vi "SE_E5_Práctica3.vi"() -> ()   [LabVIEW 2015]
uses:
  <vilib>/myRIO/Instrument Drivers/Onboard IO/DIO/typedefs/DIO Reference.ctl
  <vilib>/myRIO/Common/Instrument Driver Framework/Utilities/typedefs/myRIO Generic Hardware Reference.ctl
  <vilib>/myRIO/Common/Instrument Driver Framework/Utilities/typedefs/Hardware Version Enum.ctl
  <vilib>/myRIO/Common/Instrument Driver Framework/Utilities/typedefs/myRIO v1.0 Reference.ctl
  <vilib>/myRIO/Common/Instrument Driver Framework/Utilities/typedefs/Generic FPGA Reference.ctl
  <vilib>/myRIO/Common/Instrument Driver Framework/myRIO v1.0/DIO/typedefs/DIO Channels List.ctl
  <vilib>/myRIO/Common/Instrument Driver Framework/myRIO v1.0/DIO/typedefs/DIO Channels Enum.ctl
  <vilib>/userdefined/High Color/nirio_resource_hc.ctl
  <vilib>/myRIO/Common/Instrument Driver Framework/Utilities/vis/Is FPGA Ref Available.vi
  <vilib>/myRIO/Common/Instrument Driver Framework/myRIO v1.0/DIO/vis/myRIO v1.1 Open DIO.vi
  <vilib>/myRIO/Instrument Drivers/Onboard IO/DIO/vis/Read.vi
  <vilib>/myRIO/Common/Instrument Driver Framework/Utilities/vis/Validate Channels.vi
  <vilib>/myRIO/Common/Instrument Driver Framework/myRIO v1.0/DIO/vis/myRIO v1.0 Reserve DIO.vi
  <vilib>/myRIO/Common/Instrument Driver Framework/myRIO v1.0/Resource Manager/vis/myRIO v1.0 Reserve Channel List.vi
  <vilib>/myRIO/Common/Instrument Driver Framework/myRIO v1.0/DIO/vis/myRIO v1.0 Build MUX Configuration DIO.vi
  <vilib>/myRIO/Common/Instrument Driver Framework/myRIO v1.0/Resource Manager/vis/myRIO v1.0 Reserve Channel.vi
  <vilib>/myRIO/Common/Instrument Driver Framework/myRIO v1.0/Resource Manager/vis/myRIO v1.0 Unreserve Channel.vi
  <vilib>/myRIO/Common/Instrument Driver Framework/myRIO v1.0/Resource Manager/vis/myRIO v1.0 Create Configuration List.vi
  <vilib>/myRIO/Common/Instrument Driver Framework/myRIO v1.0/Resource Manager/vis/myRIO v1.0 Build Mutex Name.vi
  <vilib>/Utility/VariantDataType/GetNumericInfo.vi
  <vilib>/Utility/error.llb/Error Cluster From Error Code.vi
  <vilib>/myRIO/Common/Instrument Driver Framework/myRIO v1.0/myRIO v1.1 Open.vi
  <vilib>/myRIO/Common/Instrument Driver Framework/Utilities/vis/IO Manager.vi
  <vilib>/myRIO/Common/Instrument Driver Framework/Utilities/vis/Configuration Manager.vi
  <vilib>/myRIO/Common/Instrument Driver Framework/myRIO v1.0/Resource Manager/vis/myRIO v1.0 Configure IO.vi
  <vilib>/myRIO/Common/Instrument Driver Framework/myRIO v1.0/myRIO v1.0 Close.vi
  <vilib>/myRIO/Common/Instrument Driver Framework/myRIO v1.0/DIO/vis/myRIO v1.0 Read DIO.vi
  <vilib>/myRIO/Express VI/Onboard IO/DI/DI Express VI.xnode
  <vilib>/myRIO/Instrument Drivers/Onboard IO/DIO/vis/myRIO DIO Open.xnode
  <vilib>/myRIO/Express VI/Onboard IO/DO/DO Express VI.xnode
  <vilib>/myRIO/Instrument Drivers/Onboard IO/DIO/DIO.lvlib
panel:
  in  "stop":bool
  out "Q4":bool
  out "Q3":bool
  out "Q2":bool
  out "Q1":bool
  in  "I5":bool
  in  "I4":bool
  in  "I3":bool
  in  "I2":bool
  in  "I1":bool
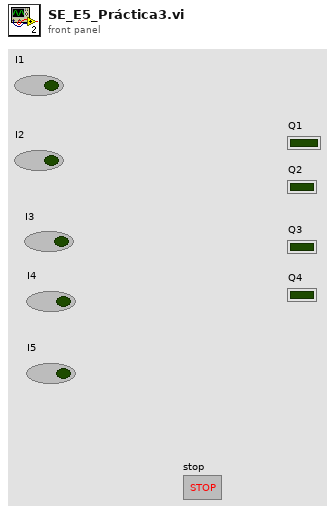
[diagram p1: front panel]
types:
  T1 = typedef "DIO.lvlib/DIO Reference.ctl" = cluster{"myRIO Reference":T2, "DIO Channels List":T6}
  T2 = typedef "myRIO Generic Hardware Reference.ctl" = cluster{"myRIO Model":T3, "myRIO Hardware Reference":T4}
  T3 = typedef "Hardware Version Enum.ctl" = enum16{"Unknown", "myRIO-1900", "myRIO-1950", "roboRIO"}
  T4 = typedef "myRIO v1.0 Reference.ctl" = cluster{"Generic FPGA Reference":T5, "Allow multiple opens":bool}
  T5 = typedef "Generic FPGA Reference.ctl" = refnum<k20>
  T6 = typedef "DIO Channels List.ctl" = T7[]
  T7 = typedef "DIO Channels Enum.ctl" = enum16{"Not Connected", "C/DIO0", "C/DIO1", "C/DIO2", "C/DIO3", "C/DIO4", "C/DIO5", "C/DIO6", "C/DIO7", "A/DIO0", "A/DIO1", "A/DIO2", "A/DIO3", "A/DIO4", "A/DIO5", "A/DIO6", "A/DIO7", "A/DIO8", "A/DIO9", "A/DIO10", "A/DIO11", "A/DIO12", "A/DIO13", "A/DIO14", "A/DIO15", "B/DIO0", "B/DIO1", "B/DIO2", "B/DIO3", "B/DIO4", "B/DIO5", "B/DIO6", "B/DIO7", "B/DIO8", "B/DIO9", "B/DIO10", "B/DIO11", "B/DIO12", "B/DIO13", "B/DIO14", "B/DIO15", "LED0", "LED1", "LED2", "LED3", "Button0", "DIO/DIO0", "DIO/DIO1", "DIO/DIO2", "DIO/DIO3", "DIO/DIO4", "DIO/DIO5", "DIO/DIO6", "DIO/DIO7", "DIO/DIO8", "DIO/DIO9", "SPI/CS0", "SPI/CS1", "SPI/CS2", "SPI/CS3", "LED RADIO (Green)", "LED RADIO (Red)", "LED COMM (Green)", "LED COMM (Red)", "LED MODE (Green)", "LED MODE (Red)"}
  T8 = typedef "nirio_resource_hc.ctl" = tag
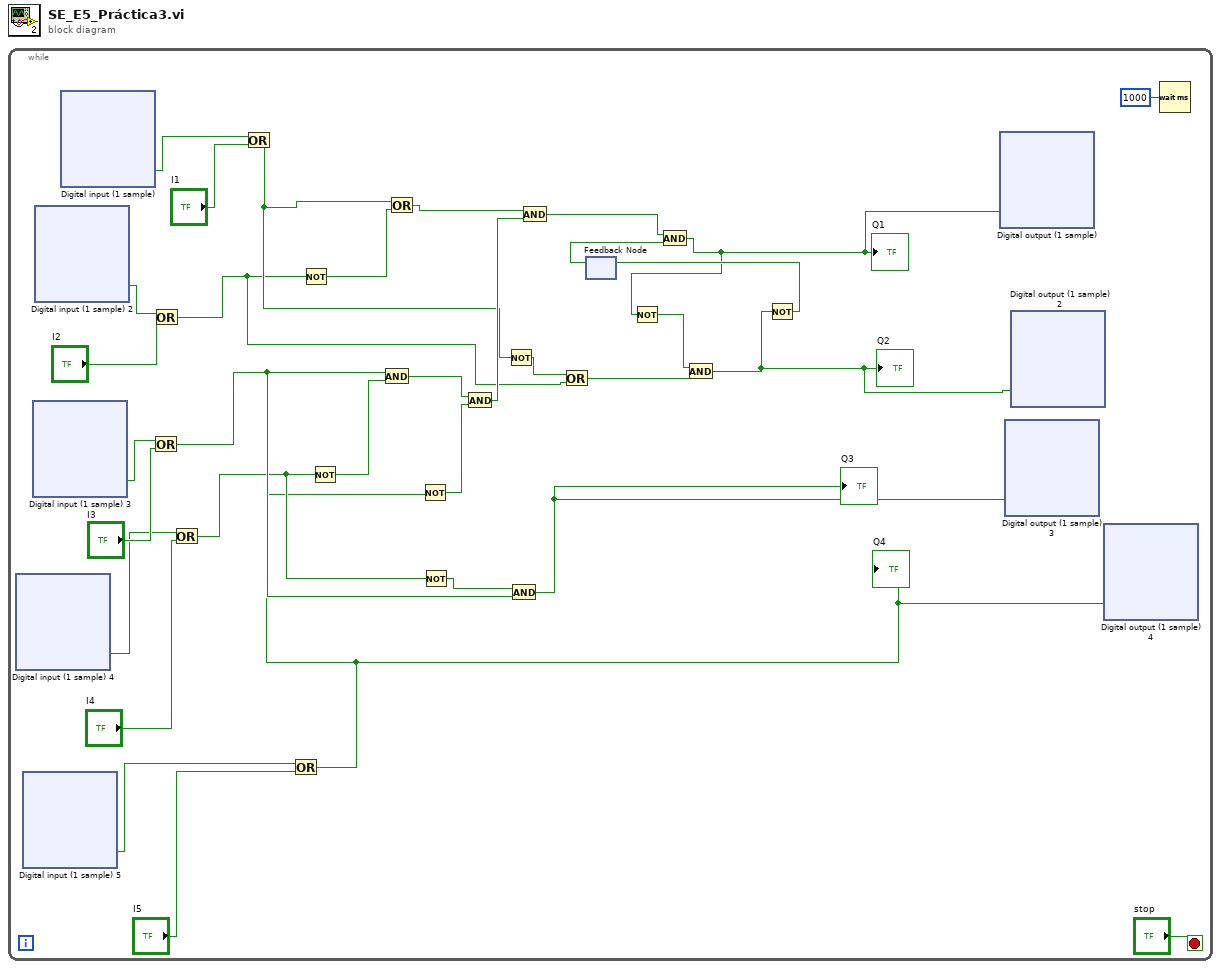
[diagram p0: block diagram]
diagram:
  n1 = while {
    stop <- "stop" stop-if-true
    n2 = xnode "Digital input (1 sample) 4"() -> ("I4 (A/DIO6 (Pin 23))"=w3:bool)  [unwired: 1 in, 1 out]
    n3 = xnode "Digital input (1 sample) 5"() -> ("I5 (A/DIO8 (Pin 27))"=w2:bool)  [unwired: 1 in, 1 out]
    n4 = xnode "Digital input (1 sample) 3"() -> ("I3 (A/DIO4 (Pin 19))"=w11:bool)  [unwired: 1 in, 1 out]
    n5 = xnode "Digital input (1 sample) 2"() -> ("I2 (A/DIO2 (Pin 15))"=w6:bool)  [unwired: 1 in, 1 out]
    n6 = xnode "Digital input (1 sample)"() -> ("I1 (A/DIO0 (Pin 11))"=w15:bool)  [unwired: 1 in, 1 out]
    n7 = Or(x=w11, y="I3") -> (x .or. y?=w12:bool)
    n8 = Or(x=w6, y="I2") -> (x .or. y?=w14:bool)
    n9 = Or(x=w3, y="I4") -> (x .or. y?=w8:bool)
    n10 = Or(x=w15, y="I1") -> (x .or. y?=w17:bool)
    n11 = Or(x=w2, y="I5") -> (x .or. y?=w1:bool)
    "Q4" <- w1
    n12 = Not(x=w14) -> (.not. x?=w33:bool)
    n13 = Not(x=w8) -> (.not. x?=w30:bool)
    n14 = And(x=w12, y=w30) -> (x .and. y?=w29:bool)
    n15 = Or(x=w17, y=w33) -> (x .or. y?=w32:bool)
    n16 = Not(x=w1) -> (.not. x?=w28:bool)
    n17 = Not(x=w8) -> (.not. x?=w21:bool)
    n18 = And(x=w29, y=w28) -> (x .and. y?=w27:bool)
    n19 = Not(x=w17) -> (.not. x?=w26:bool)
    n20 = And(x=w21, y=w12) -> (x .and. y?=w18:bool)
    "Q3" <- w18
    n21 = And(x=w32, y=w27) -> (x .and. y?=w31:bool)
    n22 = Or(x=w26, y=w14) -> (x .or. y?=w25:bool)
    n23 = feedback #1() -> (w22:bool)  [unwired: 1 in]
    n24 = And(x=w31, y=w22) -> (x .and. y?=w20:bool)
    "Q1" <- w20
    n25 = Not(x=w20) -> (.not. x?=w24:bool)
    n26 = And(x=w24, y=w25) -> (x .and. y?=w19:bool)
    "Q2" <- w19
    n27 = Not(x=w19) -> (.not. x?=w23:bool)
    n28 = feedback-in #1(w23) -> ()
    n29 = xnode "Digital output (1 sample)"("Q1\n (A/DIO1 (Pin 13))"=w20) -> ()  [unwired: 1 in, 1 out]
    n30 = xnode "Digital output (1 sample) 3"("Q3\n (A/DIO5 (Pin 21))"=w18) -> ()  [unwired: 1 in, 1 out]
    n31 = xnode "Digital output (1 sample) 2"("Q2\nQ2\nQ2\n (A/DIO3 (Pin 17))"=w19) -> ()  [unwired: 1 in, 1 out]
    n32 = xnode "Digital output (1 sample) 4"("Q4\n (A/DIO7 (Pin 25))"=w1) -> ()  [unwired: 1 in, 1 out]
    n33 = Wait (ms)(milliseconds to wait=u32 1000) -> ()  [unwired: 1 out]
  }
